vi "Log System Errors to File.vi"(8 "error out":errorcluster, 10 "Comments":string, 11 "Path":path=path "C:/Documents and Settings/Inalfa/Desktop") -> (0 "error out":errorcluster)   [LabVIEW 2018]
uses:
  <vilib>/Utility/file.llb/Read From Spreadsheet File (string).vi
  <vilib>/Utility/file.llb/Write To Spreadsheet File (string).vi
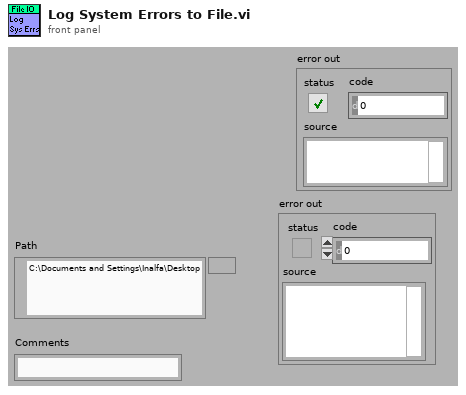
[diagram p1: front panel]
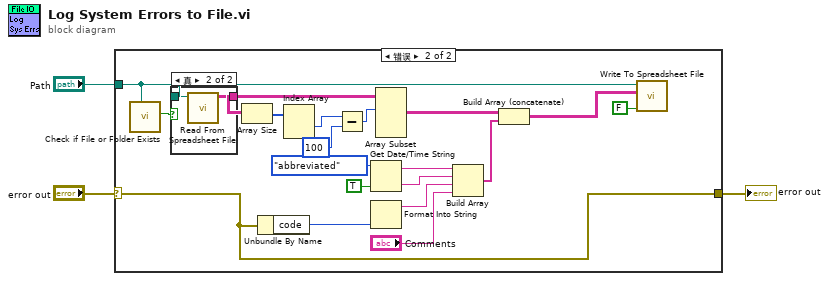
[diagram p0: block diagram]
diagram:
  n1 = case shown="错误" "error out" {
    selector: "error out" -> [w4 w17]
    tunnel: [w4 w17] -> w2
    tunnel: "Path" -> [_ w6]
    frame No Error {
    }
    frame Error {
      n2 = call <vilib>:"Check if File or Folder Exists.vi"("path"=w6) -> ("file or folder exists?"=w5:bool)  [unwired: 8 in, 2 out]
      n3 = case shown="真" w5 {
        tunnel: [_ w25] -> w13
        tunnel: w6 -> [_ w24]
        frame False {
        }
        frame True {
          n4 = call-poly <vilib>:"Read From Spreadsheet File.vi"("file path (dialog if empty)"=w24) -> ("all rows"=w25:string[][])  [unwired: 6 in, 4 out]
        }
      }
      n5 = Array Size(array=w13) -> (size(s)=w12:i32[])
      n6 = Unbundle By Name(w17) -> ("code"=w21:i32)
      n7 = Index Array(array=w12) -> (element #1=w11:i32)  [unwired: 2 in, 1 out]
      n8 = Subtract(x=w11, y=100) -> (x-y=w10:i32)
      n9 = Get Date/Time String(date format (0)=enum16{"short", "long", "abbreviated"}."abbreviated", want seconds? (F)=TRUE) -> (date string=w23:string, time string=w22:string)  [unwired: 1 out]
      n10 = Format Into String(w21) -> (resulting string=w20:string)  [unwired: 3 in, 1 out]
      n11 = Array Subset(array=w13, index (row)=w10) -> (w15:string[][])  [unwired: 3 in]
      n12 = Build Array(w23, w22, w20, "Comments") -> (w16:string[])
      n13 = Build Array (concatenate)(w15, w16) -> (w14:string[][])
      n14 = call-poly <vilib>:"Write To Spreadsheet File.vi"("append to file? (new file:F)"=FALSE, "2D data"=w14, "file path (dialog if empty)"=w6) -> ()  [unwired: 3 in, 3 out]
    }
  }
  "error out" <- w2
